vi "WS1050_Extract Data From Scope_60_95 Amp.vi"(0 "file path":path=path "S:/_Employee_Folders/Andy temp/SN01/444AB_04__SN01_C1_S1_UP_Switch_Time_data.csv", 1 "60% Amp":dbl=0.6, 2 "95% Amp":dbl=0.95, 5 "Noise Level(V)":dbl=0.005, 9 "End point":i32=4000, 11 "error in (no error)":errorcluster, 12 "90% Amp":dbl=0.9) -> (3 "AMP(v)":dbl=1.1, 4 "Amp(mv)":string, 6 "T2(us)":string, 8 "T3(us)":string, 10 "T1(us)":string, 15 "error out":errorcluster)   [LabVIEW 2012]
uses:
  <vilib>/Utility/file.llb/Read From Spreadsheet File (string).vi
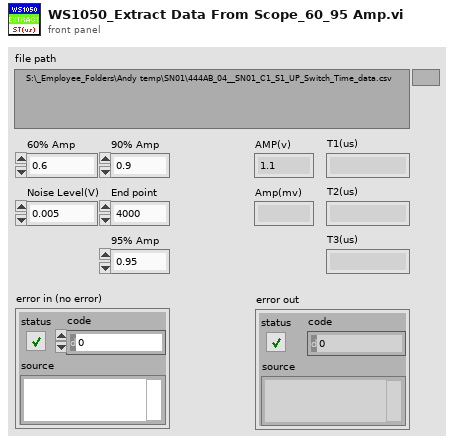
[diagram p1: front panel]
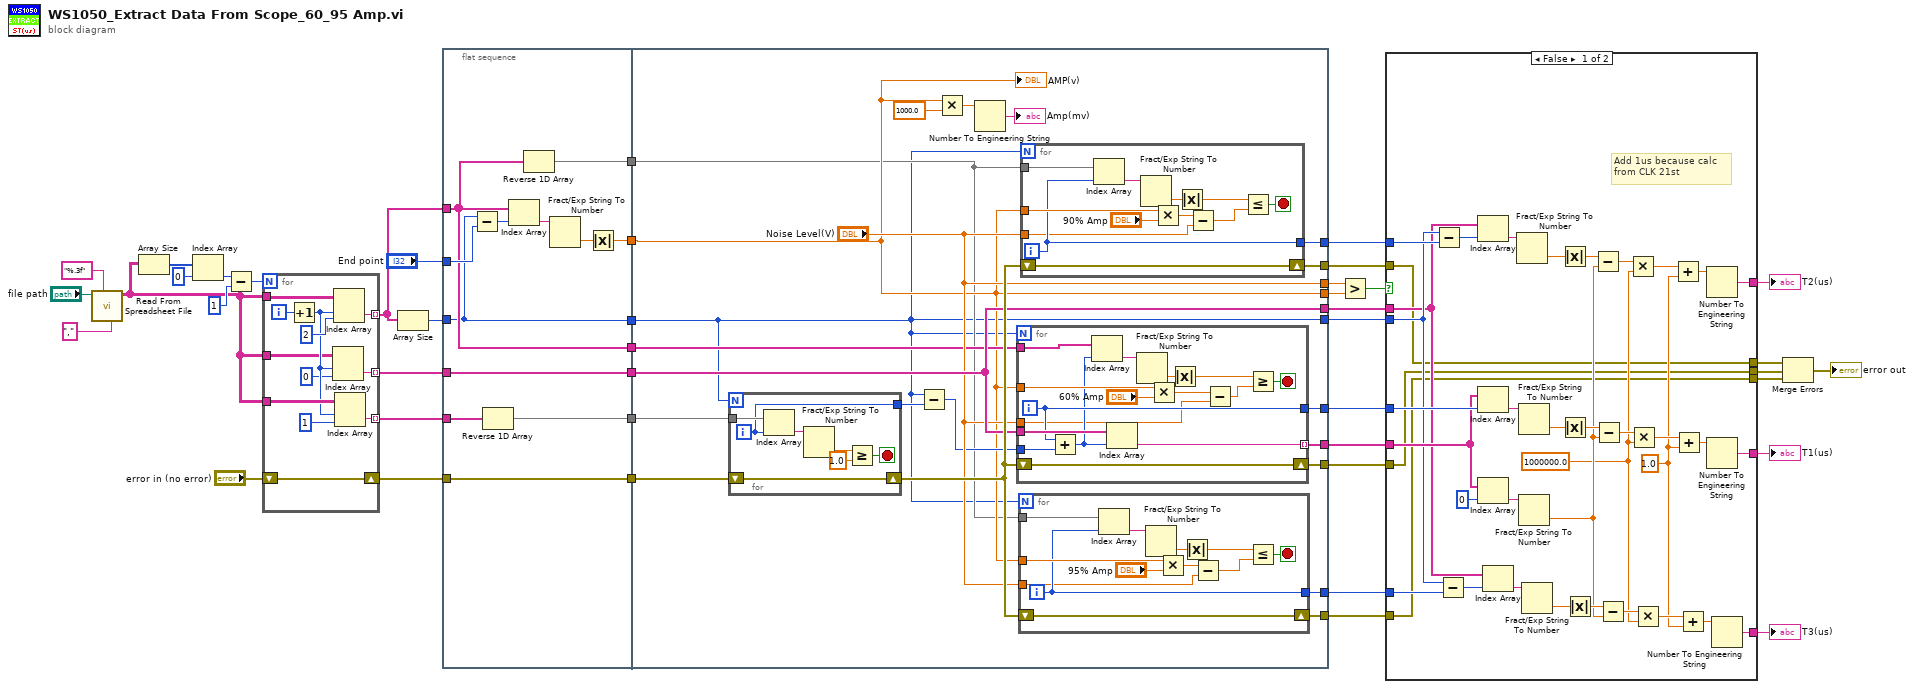
[diagram p0: block diagram]
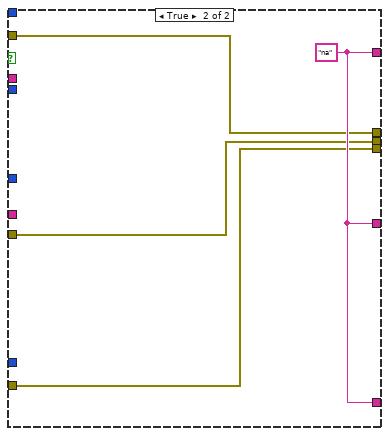
[diagram p2: hidden frame]
diagram:
  n1 = call-poly <vilib>:"Read From Spreadsheet File.vi"("delimiter (\\t)"="," ("delimiter (\\t)"), "format (%s)"="%.3f" ("format (%.3f)"), "file path (dialog if empty)"="file path") -> ("all rows"=w23:string[][])  [unwired: 4 in, 4 out]
  n2 = Array Size(array=w23) -> (size(s)=w39:i32[])
  n3 = Index Array(array=w39, index=0) -> (element=w37:i32)
  n4 = Subtract(x=w37, y=1) -> (x-y=w24:i32)
  n5 = for {
    N: w24 -> [_]
    tunnel: w23 -> [w54]
    tunnel: [w51] -> w7 mode=indexing
    tunnel: w23 -> [w50]
    tunnel: [w48] -> w34 mode=indexing
    tunnel: w23 -> [w46]
    tunnel: [w44] -> w25 mode=indexing
    shift-right: [w43] -> w32
    shift-left: "error in (no error)" -> [w43]
    i -> [w52]
    n6 = Increment(x=w52) -> (x+1=w47:i32)
    n7 = Index Array(array=w46, index (row)=w47, index (col)=0 ("disabled index (col)")) -> (element=w44:string)
    n8 = Index Array(array=w54, index (row)=w47, index (col)=2 ("disabled index (col)")) -> (element=w51:string)
    n9 = Index Array(array=w50, index (row)=w47, index (col)=1 ("disabled index (col)")) -> (element=w48:string)
  }
  n10 = Array Size(array=w7) -> (size(s)=w6:i32)
  n11 = flat-sequence {
    tunnel: "End point" -> [w61]
    tunnel: w25 -> [w65]
    tunnel: w32 -> [w66]
    tunnel: w34 -> [w59]
    tunnel: [w66] -> w9
    tunnel: [w65] -> w8
    tunnel: w7 -> [w56]
    tunnel: w6 -> [w55]
    tunnel: [w60] -> w5
    tunnel: [w58] -> w4
    tunnel: [w57] -> w3
    tunnel: [w56] -> w2
    tunnel: [w55] -> w1
    tunnel: [w87] -> w35
    tunnel: [w85] -> w30
    tunnel: [w84] -> w29
    tunnel: [w80] -> w27
    tunnel: [w79] -> w26
    tunnel: [w67] -> w19
    tunnel: [w74] -> w18
    tunnel: [w76] -> w22
    tunnel: [w75] -> w20
    tunnel: ["Noise Level(V)"] -> w16
    tunnel: [w70] -> w15
    tunnel: w9 -> [w86]
    tunnel: w8 -> [w74]
    tunnel: w5 -> [w70]
    tunnel: w4 -> [w69]
    tunnel: w3 -> [w68]
    tunnel: w2 -> [w71]
    tunnel: w1 -> [w67]
    frame #0 {
      n12 = Subtract(x=w55, y=w61) -> (x-y=w64:i32)
      n13 = Reverse 1D Array(array=w59) -> (reversed array=w58:string[])
      n14 = Index Array(array=w56, index=w64) -> (element=w62:string)
      n15 = Reverse 1D Array(array=w56) -> (reversed array=w57:string[])
      n16 = Fract/Exp String To Number(string=w62) -> (number=w63:dbl)  [unwired: 3 in, 1 out]
      n17 = Absolute Value(x=w63) -> (abs(x)=w60:dbl)
    }
    frame #1 {
      n18 = for {
        N: w67 -> [_]
        tunnel: w69 -> [w134]
        tunnel: [w131] -> w78
        shift-right: [w129] -> w77
        shift-left: w86 -> [w129]
        i -> [w131]
        stop <- w132 stop-if-true
        n19 = Index Array(array=w134, index=w131) -> (element=w128:string)
        n20 = Fract/Exp String To Number(string=w128) -> (number=w130:dbl)  [unwired: 3 in, 1 out]
        n21 = Greater Or Equal?(x=w130, y=1.0) -> (x >= y?=w132:bool)
      }
      n22 = Subtract(x=w67, y=w78) -> (x-y=w72:i32)
      n23 = Multiply(x=w70, y=1000.0) -> (x*y=w82:dbl)
      n24 = Number To Engineering String(4:w82) -> (0:→"Amp(mv)":string)  [unwired: 3 in]
      n25 = for {
        N: w67 -> [_]
        tunnel: w71 -> [w127]
        tunnel: w70 -> [w125]
        tunnel: w74 -> [w124]
        tunnel: [w123] -> w79 mode=indexing
        tunnel: [w120] -> w87
        tunnel: w72 -> [w122]
        shift-right: [w117] -> w84
        shift-left: w77 -> [w117]
        tunnel: "Noise Level(V)" -> [w112]
        i -> [w120]
        stop <- w126 stop-if-true
        n26 = Add(x=w120, y=w122) -> (x+y=w119:i32)
        n27 = Index Array(array=w127, index=w119) -> (element=w121:string)
        n28 = Index Array(array=w124, index=w119) -> (element=w123:string)
        n29 = Fract/Exp String To Number(string=w121) -> (number=w116:dbl)  [unwired: 3 in, 1 out]
        n30 = Multiply(x=w125, y="60% Amp") -> (x*y=w113:dbl)
        n31 = Absolute Value(x=w116) -> (abs(x)=w115:dbl)
        n32 = Subtract(x=w113, y=w112) -> (x-y=w114:dbl)
        n33 = Greater Or Equal?(x=w115, y=w114) -> (x >= y?=w126:bool)
      }
      n34 = for {
        N: w67 -> [_]
        tunnel: w68 -> [w99]
        tunnel: w70 -> [w97]
        tunnel: [w93] -> w75
        shift-right: [w95] -> w76
        shift-left: w77 -> [w95]
        tunnel: "Noise Level(V)" -> [w88]
        i -> [w93]
        stop <- w98 stop-if-true
        n35 = Index Array(array=w99, index=w93) -> (element=w92:string)
        n36 = Fract/Exp String To Number(string=w92) -> (number=w94:dbl)  [unwired: 3 in, 1 out]
        n37 = Multiply(x=w97, y="95% Amp") -> (x*y=w90:dbl)
        n38 = Absolute Value(x=w94) -> (abs(x)=w91:dbl)
        n39 = Subtract(x=w90, y=w88) -> (x-y=w89:dbl)
        n40 = Less Or Equal?(x=w91, y=w89) -> (x <= y?=w98:bool)
      }
      n41 = for {
        N: w67 -> [_]
        tunnel: w68 -> [w111]
        tunnel: w70 -> [w109]
        tunnel: [w105] -> w80
        shift-right: [w107] -> w85
        shift-left: w77 -> [w107]
        tunnel: "Noise Level(V)" -> [w100]
        i -> [w105]
        stop <- w110 stop-if-true
        n42 = Index Array(array=w111, index=w105) -> (element=w104:string)
        n43 = Fract/Exp String To Number(string=w104) -> (number=w106:dbl)  [unwired: 3 in, 1 out]
        n44 = Multiply(x=w109, y="90% Amp") -> (x*y=w102:dbl)
        n45 = Absolute Value(x=w106) -> (abs(x)=w103:dbl)
        n46 = Subtract(x=w102, y=w100) -> (x-y=w101:dbl)
        n47 = Less Or Equal?(x=w103, y=w101) -> (x <= y?=w110:bool)
      }
      "AMP(v)" <- w70
    }
  }
  n48 = Greater?(x=w16, y=w15) -> (0:w17:bool)
  n49 = case shown="False" w17 {
    tunnel: w35 -> [w168 _]
    tunnel: [w166 w175] -> w31
    tunnel: w30 -> [w137 w174]
    tunnel: w29 -> [w136 w173]
    tunnel: [w165 w175] -> w28
    tunnel: w27 -> [w154 _]
    tunnel: w26 -> [w153 _]
    tunnel: w22 -> [w135 w172]
    tunnel: [w144 w175] -> w21
    tunnel: w20 -> [w143 _]
    tunnel: w19 -> [w142 _]
    tunnel: w18 -> [w141 _]
    tunnel: [w137 w174] -> w14
    tunnel: [w136 w173] -> w13
    tunnel: [w135 w172] -> w12
    frame False {
      w138 = 1.0 ("y")
      w139 = 1000000.0 ("y")
      # "Add 1us because calc \nfrom CLK 21st"
      n50 = Subtract(x=w142, y=w154) -> (x-y=w152:i32)
      n51 = Subtract(x=w142, y=w143) -> (x-y=w151:i32)
      n52 = Index Array(array=w141, index=w152) -> (element=w163:string)
      n53 = Index Array(array=w153, index=w168) -> (element=w171:string)
      n54 = Index Array(array=w153, index=0) -> (element=w169:string)
      n55 = Index Array(array=w141, index=w151) -> (element=w146:string)
      n56 = Fract/Exp String To Number(string=w163) -> (number=w157:dbl)  [unwired: 3 in, 1 out]
      n57 = Fract/Exp String To Number(string=w171) -> (number=w155:dbl)  [unwired: 3 in, 1 out]
      n58 = Fract/Exp String To Number(string=w169) -> (number=w140:dbl)  [unwired: 3 in, 1 out]
      n59 = Fract/Exp String To Number(string=w146) -> (number=w150:dbl)  [unwired: 3 in, 1 out]
      n60 = Absolute Value(x=w157) -> (abs(x)=w158:dbl)
      n61 = Absolute Value(x=w155) -> (abs(x)=w156:dbl)
      n62 = Absolute Value(x=w150) -> (abs(x)=w149:dbl)
      n63 = Subtract(x=w158, y=w140) -> (x-y=w164:dbl)
      n64 = Subtract(x=w156, y=w140) -> (x-y=w167:dbl)
      n65 = Subtract(x=w149, y=w140) -> (x-y=w145:dbl)
      n66 = Multiply(x=w164, y=w139) -> (x*y=w159:dbl)
      n67 = Multiply(x=w167, y=w139) -> (x*y=w161:dbl)
      n68 = Multiply(x=w145, y=w139) -> (x*y=w148:dbl)
      n69 = Add(x=w159, y=w138) -> (x+y=w160:dbl)
      n70 = Add(x=w161, y=w138) -> (x+y=w162:dbl)
      n71 = Add(x=w148, y=w138) -> (x+y=w147:dbl)
      n72 = Number To Engineering String(4:w160) -> (0:w165:string)  [unwired: 3 in]
      n73 = Number To Engineering String(4:w162) -> (0:w166:string)  [unwired: 3 in]
      n74 = Number To Engineering String(4:w147) -> (0:w144:string)  [unwired: 3 in]
    }
    frame True {
      w175 = "na"
    }
  }
  "T1(us)" <- w31
  "T2(us)" <- w28
  "T3(us)" <- w21
  n75 = Merge Errors(w14, w13, w12) -> (→"error out":errorcluster)
